vi "Convert Dictionary to ITEMs and VALUEs.vi"(8 "error in (no error)":errorcluster, 11 "Data (Dictionary)":T1[](array[typedef])) -> (0 "error out":errorcluster, 1 "2D Array of Variants":variant[][](array[variant]), 2 "ITEMS":string[](array[string]), 3 "Data (Dictionary)":T1[](array[typedef]))   [LabVIEW 2019, in "LV-Data.PGSQL.lvclass"]
uses:
  LV-Data.PGSQL.lvclass
  <userlib>/LevyLab/LV-Data/LV-Data/Typedefs/Dictionary--cluster.ctl
  <userlib>/LevyLab/LV-Data/LV-Data/LV-Data.lvclass
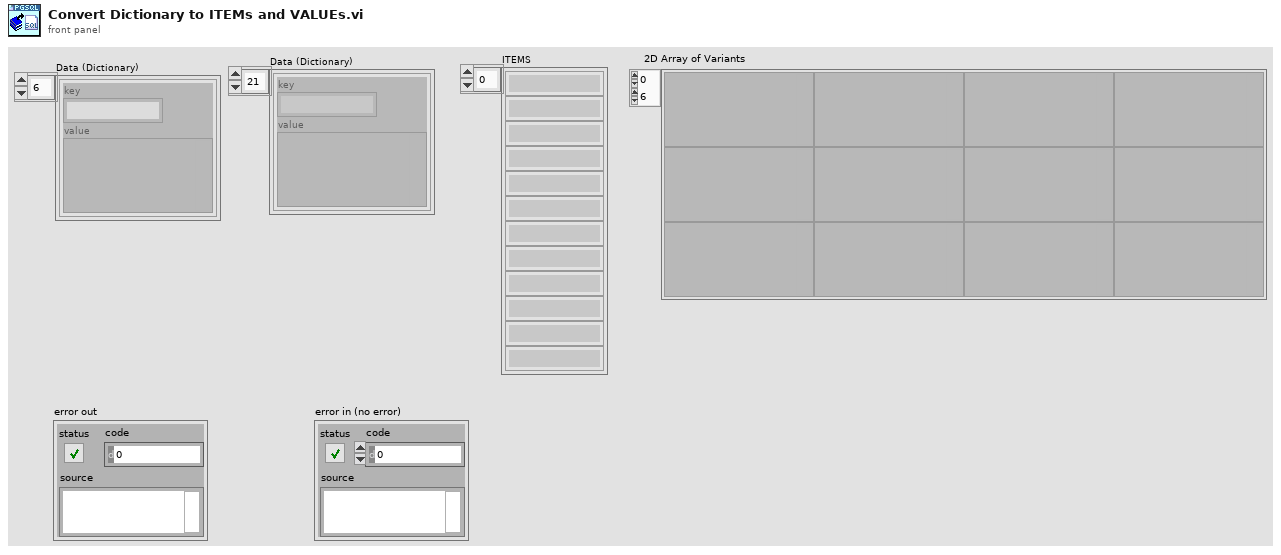
[diagram p1: front panel]
types:
  T1 = typedef "LV-Data.lvclass/Dictionary--cluster.ctl" = cluster{"key":string, "value":variant}
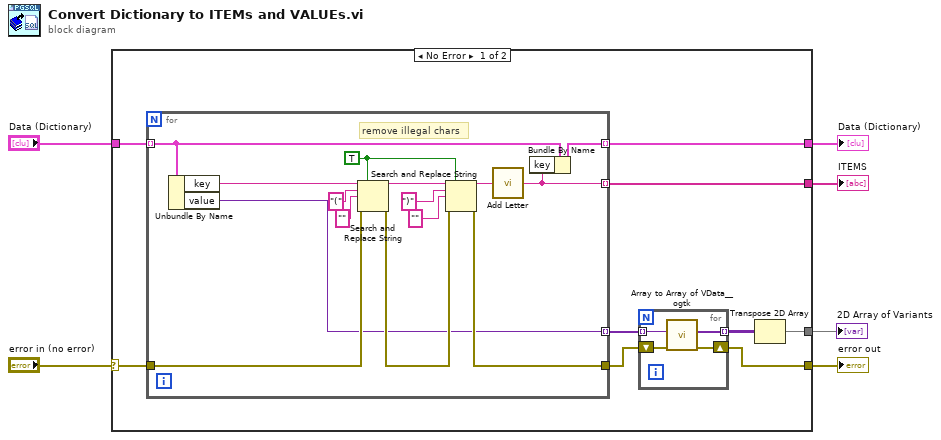
[diagram p0: block diagram]
diagram:
  n1 = case shown="No Error" "error in (no error)" {
    selector: "error in (no error)" -> [w14 w35]
    tunnel: [w7 w35] -> w6
    tunnel: "Data (Dictionary)" -> [w15 _]
    tunnel: [w13 _] -> w3
    tunnel: [w12 _] -> w2
    tunnel: [w9 _] -> w1
    frame No Error {
      n2 = for {
        tunnel: w15 -> [w20] mode=indexing
        tunnel: w14 -> [w28]
        tunnel: [w19] -> w8
        tunnel: [w21] -> w13 mode=indexing
        tunnel: [w16] -> w12 mode=indexing
        tunnel: [w18] -> w10 mode=indexing
        w23 = TRUE ("replace all? (F)")
        # "remove illegal chars"
        n3 = Unbundle By Name(w20) -> ("key"=w29:string, "value"=w18:variant)
        n4 = Search and Replace String(replace all?=w23, input string=w29, search string="(", replace string="" ("replace string (\"\")"), error in=w28) -> (result string=w24:string, error out=w22:errorcluster)  [unwired: 3 in, 2 out]
        n5 = Search and Replace String(replace all?=w23, input string=w24, search string=")", replace string="" ("replace string (\"\")"), error in=w22) -> (result string=w17:string, error out=w19:errorcluster)  [unwired: 3 in, 2 out]
        n6 = call <userlib>:"Add Letter.vi"("string"=w17) -> ("result string"=w16:string)
        n7 = Bundle By Name(cluster=w20, "key"=w16) -> (w21:T1)
      }
      n8 = for {
        tunnel: [w34] -> w11 mode=indexing
        tunnel: w10 -> [w33] mode=indexing
        shift-right: [w31] -> w7
        shift-left: w8 -> [w32]
        n9 = call <userlib>:"Array to Array of VData__ogtk.vi"("error in (no error)"=w32, "MultiD Array"=w33) -> ("error out"=w31:errorcluster, "1D Array of Variants"=w34:variant[])  [unwired: 8 in]
      }
      n10 = Transpose 2D Array(2D array=w11) -> (transposed array=w9:variant[][])
    }
    frame Error {
    }
  }
  "ITEMS" <- w2
  "error out" <- w6
  "Data (Dictionary)" <- w3
  "2D Array of Variants" <- w1
